vi "publishMonoId.vi"(8 "error in (no error)":errorcluster, 10 "monoId":string, 11 "MonoCommunicator in":refnum<class "MonoCommunicator.lvclass">) -> (0 "error out":errorcluster, 3 "MonoCommunicator out":refnum<class "MonoCommunicator.lvclass">)   [LabVIEW 2016, in "MonoCommunicator.lvclass"]
uses:
  MonoCommunicator.lvclass
  Typedefs/publishers.ctl
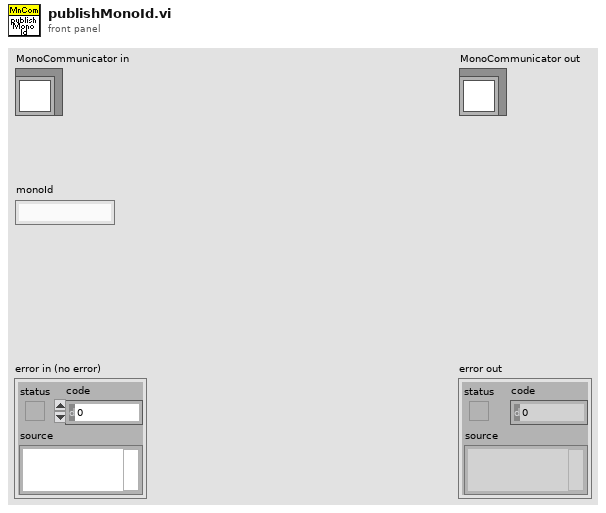
[diagram p1: front panel]
types:
  T1 = typedef "publishers.ctl" = enum16{"Wavelength", "Grating", "FrontEntranceSlitPosition", "FrontExitSlitPosition", "SoftwareStatus", "MonochromatorId"}
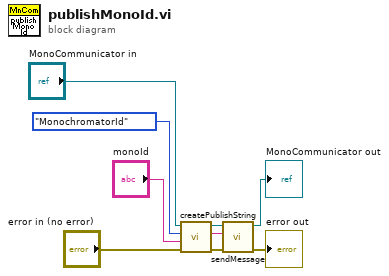
[diagram p0: block diagram]
diagram:
  n1 = call "createPublishString.vi"("error in (no error)"="error in (no error)", "parameter"="monoId", "publishers"=publishers."MonochromatorId", "MonoCommunicator in"="MonoCommunicator in") -> ("error out"=w9:errorcluster, "string"=w8:string, "MonoCommunicator out"=w7:refnum<class "MonoCommunicator.lvclass">)  [unwired: 5 in]
  n2 = call "sendMessage.vi"("error in (no error)"=w9, "message"=w8, "MonoCommunicator in"=w7) -> ("error out"=→"error out":errorcluster, "MonoCommunicator out"=→"MonoCommunicator out":refnum<class "MonoCommunicator.lvclass">)  [unwired: 7 in]
